vi "load data.vi"(8 "error in":errorcluster) -> (0 "error out":errorcluster, 3 "Array":T1[](array[typedef]))   [LabVIEW 2015]
uses:
  Controls/User data.ctl
  <vilib>/Utility/file.llb/Read Delimited Spreadsheet (string).vi
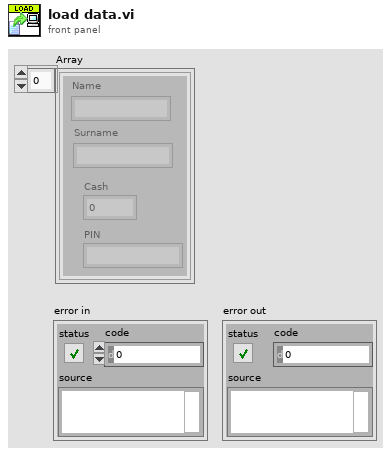
[diagram p1: front panel]
types:
  T1 = typedef "User data.ctl" = cluster{"Name":string, "Surname":string, "Cash":i32, "PIN":string}
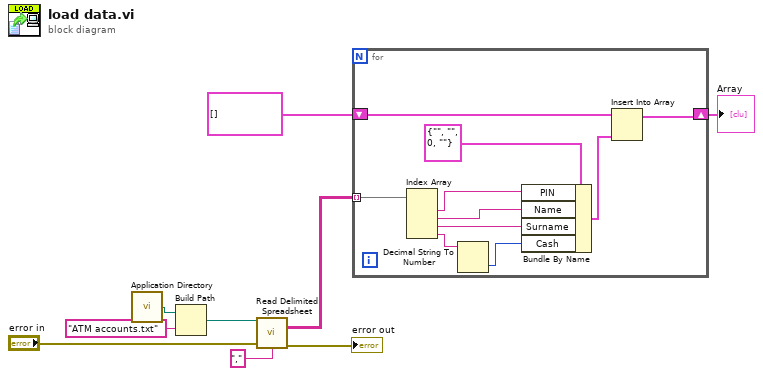
[diagram p0: block diagram]
diagram:
  n1 = call <vilib>:"Application Directory.vi"() -> ("Application Directory"=w3:path)
  n2 = Build Path(base path=w3, name or relative path="ATM accounts.txt") -> (appended path=w5:path)
  n3 = call-poly <vilib>:"Read Delimited Spreadsheet.vi"("file path (dialog if empty)"=w5, "error in (no error)"="error in", "delimiter (\\t)"="," ("delimiter (\\t)")) -> ("all rows"=w7:string[][], "error out"=→"error out":errorcluster)  [unwired: 7 in, 4 out]
  n4 = for {
    tunnel: w7 -> [w19] mode=indexing
    shift-right: [w11] -> w9
    shift-left: T1[] [] -> [w13]
    n5 = Index Array(array=w19) -> (element #1=w10:string, element #2=w14:string, element #3=w15:string, element #4=w17:string)  [unwired: 4 in]
    n6 = Decimal String To Number(string=w17) -> (number=w16:i32)  [unwired: 2 in, 1 out]
    n7 = Bundle By Name(cluster=T1 {"Name"="", "Surname"="", "Cash"=0, "PIN"=""} ("User data"), "PIN"=w10, "Name"=w14, "Surname"=w15, "Cash"=w16) -> (w12:T1)
    n8 = Insert Into Array(array=w13, new element=w12) -> (w11:T1[])  [unwired: 1 in]
  }
  "Array" <- w9
